vi "S2C_FORNAX_Proc_Globals.vi"() -> ()   [LabVIEW 2015]
panel:
  in  "Version":i32(ring)=1 items=["Fornax1"=1, "Fornax2"=2, "Fornax3"=3]
  in  "Fornax3":string
  in  "Fornax2":string
  in  "Fornax1":string
  in  "Port":i32
  in  "ClearDDS":bool
  out "AlarmQ":refnum<queue>
  in  "CmdsPath":path
  in  "Partition":string
  in  "Command":string
  in  "FnxTypes":string[][][](array[string])
  in  "FnxCmds":string[][][](array[string])
  in  "VI_Ref":refnum<vi>
  out "Refs":string[][](array[string])
  out "Response?":bool
  out "Request?":bool
  in  "RspMsg":string
  in  "ReqMsg":string
  in  "DDS_Msg":string[](array[string])
  in  "Viper_Msg":string[](array[string])
  out "FNX_Ref":refnum<k5>
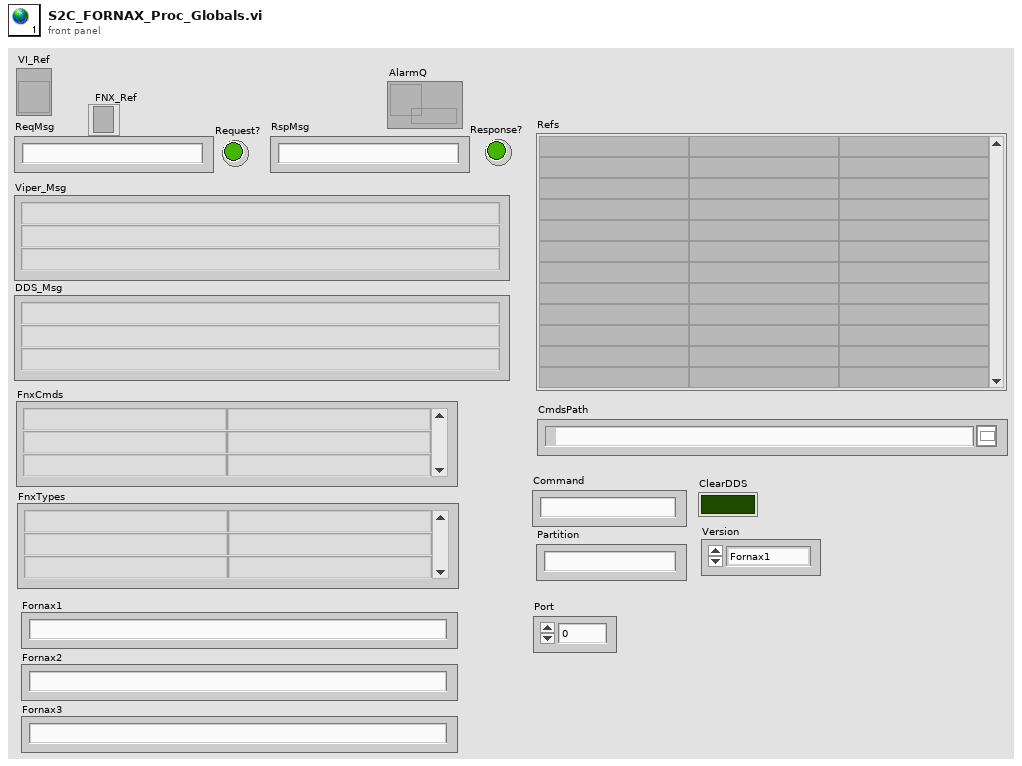
[diagram p1: front panel]
diagram:
